vi "Stop by ID.vi"(8 "Module ID":i32, 10 "Library Selected":string, 11 "References Map":map{string, refnum<vi>}(c390)) -> (0 "error out":errorcluster)   [LabVIEW 2020, in "Dashboard.lvlib"]
uses:
  Dashboard.lvlib
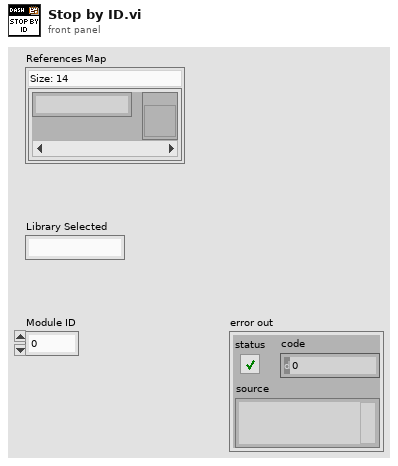
[diagram p1: front panel]
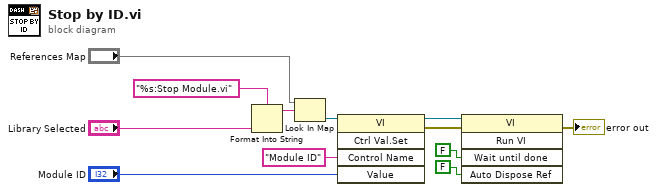
[diagram p0: block diagram]
diagram:
  n1 = Format Into String(format string="%s:Stop Module.vi", "Library Selected") -> (resulting string=w6:string)  [unwired: 2 in, 1 out]
  n2 = Look In Map(map="References Map", key=w6) -> (value=w4:refnum<vi>)  [unwired: 1 in, 1 out]
  n3 = invoke class="VI" method="Ctrl Val.Set"(reference=w4, "Control Name"="Module ID", "Value"="Module ID") -> (reference out=w1:refnum<vi>, error out=w11:errorcluster)  [unwired: 2 in, 3 out]
  n4 = invoke class="VI" method="Run VI"(reference=w1, error in=w11, "Wait until done"=FALSE ("Wait Until Done"), "Auto Dispose Ref"=FALSE ("Auto Dispose Reference")) -> (error out=→"error out":errorcluster)  [unwired: 1 in, 4 out]
